vi "OnToggleSingleplayer.vi"(8 "error in (no error)":errorcluster, 11 "Game in":refnum<class "Game.lvclass">) -> (0 "error out":errorcluster, 3 "Game out":refnum<class "Game.lvclass">)   [LabVIEW 2019, in "RT_Game.lvlib" / "Game.lvclass"]
uses:
  Game.lvclass
  Menu/States.ctl
  Game.lvclass/Game.ctl
  GameMenu/GameMenu.lvclass/GameMenu.ctl
  GameObject/GameObject.lvclass/GameObject.ctl
  GameMenu/Write ResumeBlocked.vi
  GameObject/Write IsActive.vi
  RT_Sprite/RT_Sprite.lvclass
  C:/Users/FreshBob/Dropbox/VIs/myRIO_GameConsole/RT/RT_Game/GameObject/GameObject.lvclass
  GameMenu/GameMenu.lvclass
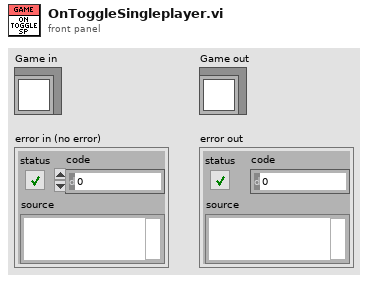
[diagram p1: front panel]
types:
  T1 = typedef "RT_Game.lvlib/Game.lvclass/States.ctl" = enum16{"Init", "Restart", "Menu", "Game", "Resume", "ToggleSingleplayer", "LoadNextGame", "ExitToMenu", "NewHighscore", "GameOver", "SlideOut"}
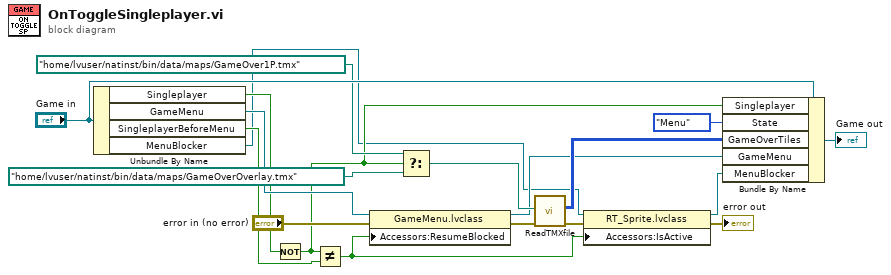
[diagram p0: block diagram]
diagram:
  n1 = Unbundle By Name("Game in") -> ("Singleplayer"=w7:bool, "GameMenu"=w9:refnum<class "GameMenu.lvclass">, "SingleplayerBeforeMenu"=w6:bool, "MenuBlocker"=w3:refnum<class "RT_Sprite.lvclass">)
  n2 = Not(x=w7) -> (.not. x?=w5:bool)
  n3 = Not Equal?(x=w5, y=w6) -> (x != y?=w1:bool)
  n4 = property class="GameMenu.lvclass"(reference=w9, error in="error in (no error)", "Accessors:ResumeBlocked"=w1) -> (reference out=w8:refnum<class "GameMenu.lvclass">, error out=w10:errorcluster)
  n5 = Select(t=path "/home/lvuser/natinst/bin/data/maps/GameOver1P.tmx" ("path to tmx-file (created with Tiles2D)"), s=w5, f=path "/home/lvuser/natinst/bin/data/maps/GameOverOverlay.tmx") -> (s? t:f=w14:path)
  n6 = call "ReadTMXfile.vi"("error in (no error)"=w10, "path to tmx-file (created with Tiles2D)"=w14) -> ("error out"=w18:errorcluster, "Tilenumbers"=w11:u32[][])  [unwired: 8 in]
  n7 = property class="RT_Sprite.lvclass"(reference=w3, error in=w18, "Accessors:IsActive"=w1) -> (reference out=w2:refnum<class "RT_Sprite.lvclass">, error out=→"error out":errorcluster)
  n8 = Bundle By Name(cluster="Game in", "Singleplayer"=w5, "State"=States."Menu", "GameOverTiles"=w11, "GameMenu"=w8, "MenuBlocker"=w2) -> (→"Game out":refnum<class "Game.lvclass">)
